vi "getPiezowaveformarray.vi"(7 "sawtooth or zigzag":bool, 8 "pixel.num":i32=10000, 9 "frames.per.z.cycle":dbl=15.0, 10 "total.z.distance":dbl=100.0, 11 "piezo scale factor":dbl=0.025) -> (3 "Array":dbl[](array[numeric]))   [LabVIEW 2017]
doc: "SciScan 1.2 160622"
uses:
  GFG/GFGnumericGet.vi
  GFG/GFG library.lvlib
panel:
  out "Waveform Graph":dbl[](graph)
  out "min value":dbl
  out "max value":dbl
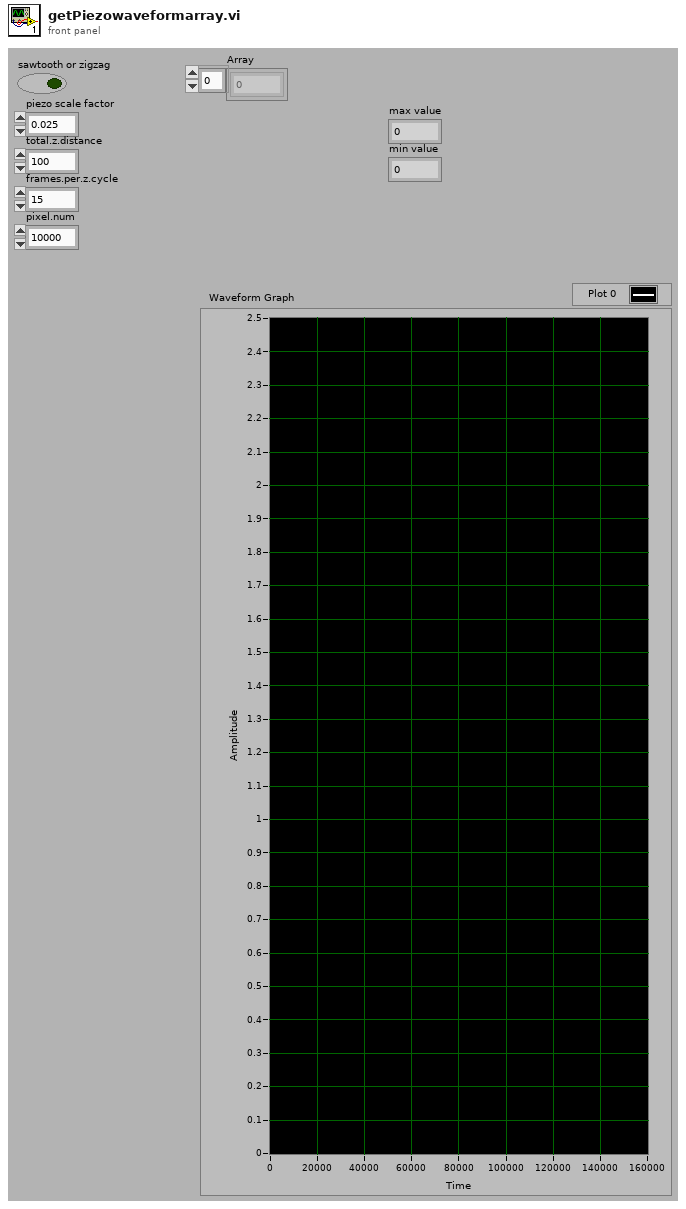
[diagram p1: front panel]
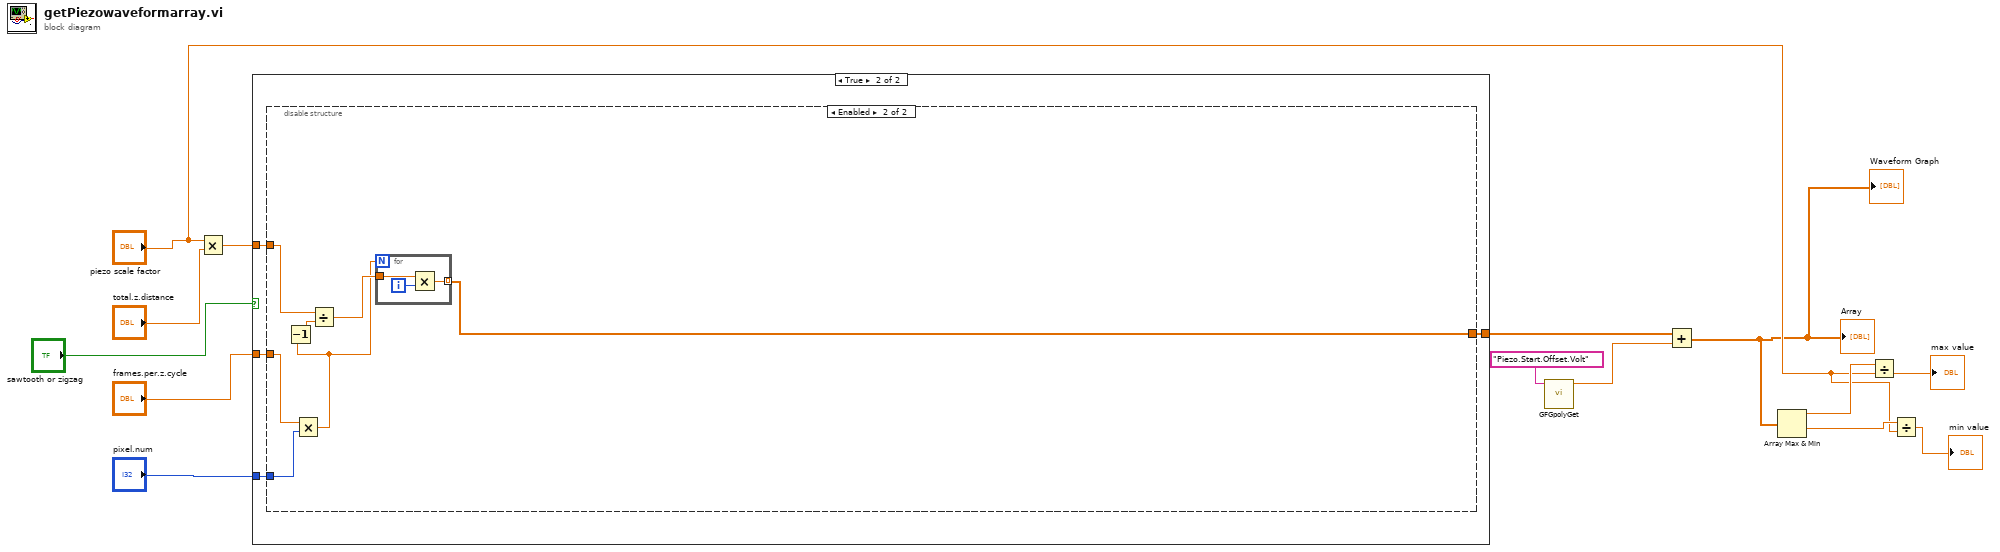
[diagram p0: block diagram]
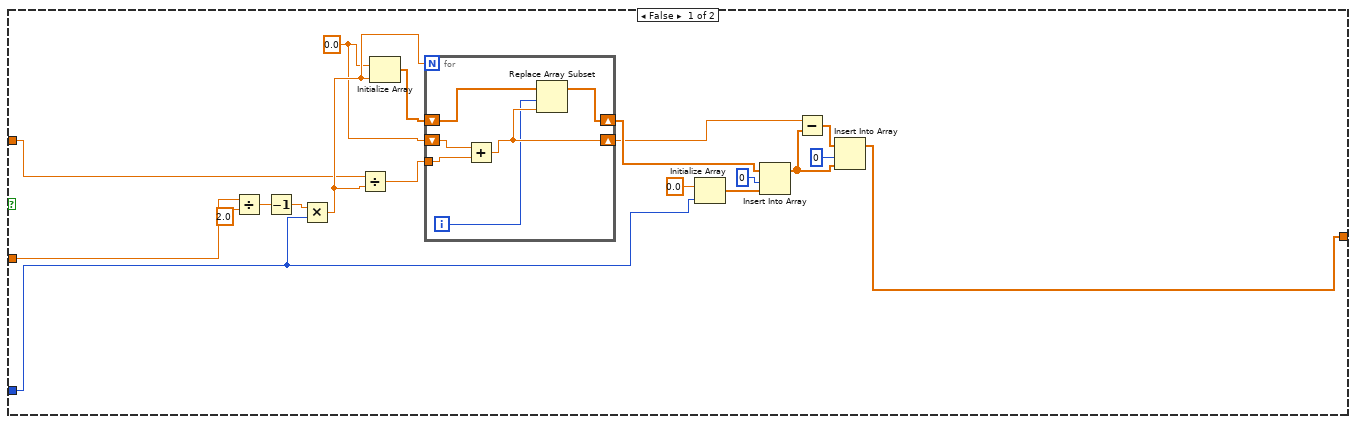
[diagram p2: hidden frame]
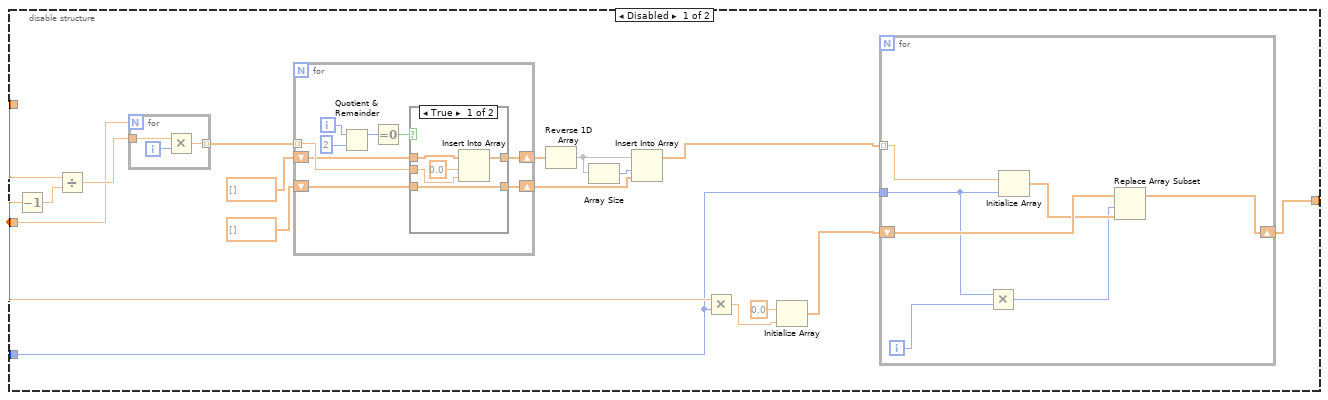
[diagram p3: hidden frame]
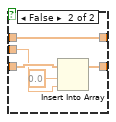
[diagram p4: hidden frame]
diagram:
  n1 = Multiply(x="piezo scale factor", y="total.z.distance") -> (x*y=w13:dbl)
  n2 = case shown="True" "sawtooth or zigzag" {
    tunnel: [w15 w43] -> w4
    tunnel: w13 -> [w18 w42]
    tunnel: "frames.per.z.cycle" -> [w17 w41]
    tunnel: "pixel.num" -> [w16 w40]
    frame False {
      w27 = 0.0 ("element")
      n3 = Divide(x=w17, y=2.0) -> (x/y=w32:dbl)
      n4 = Decrement(x=w32) -> (x-1=w31:dbl)
      n5 = Multiply(x=w31, y=w16) -> (x*y=w28:dbl)
      n6 = Divide(x=w18, y=w28) -> (x/y=w29:dbl)
      n7 = Initialize Array(w27, w28) -> (w30:dbl[])
      n8 = for {
        N: w28 -> [_]
        shift-right: [w36] -> w20
        shift-left: w30 -> [w37]
        tunnel: w29 -> [w38]
        shift-right: [w35] -> w19
        shift-left: w27 -> [w39]
        i -> [w34]
        n9 = Add(x=w39, y=w38) -> (x+y=w35:dbl)
        n10 = Replace Array Subset(array=w37, new element=w35, index=w34) -> (w36:dbl[])
      }
      n11 = Initialize Array(0.0 ("element"), w16) -> (w22:dbl[])
      n12 = Insert Into Array(array=w20, index=0, new element=w22) -> (w26:dbl[])
      n13 = Subtract(x=w19, y=w26) -> (x-y=w25:dbl[])
      n14 = Insert Into Array(array=w25, index=0, new element=w26) -> (w15:dbl[])
    }
    frame True {
      n15 = disable-structure shown="Enabled" {
        disable-tunnel: [w48 w90] -> w43
        disable-tunnel: w42 -> [w47 w95]
        disable-tunnel: w41 -> [w46 w94]
        disable-tunnel: w40 -> [w45 w93]
        frame Disabled {
          n16 = Decrement(x=w46) -> (x-1=w44:dbl)
          n17 = Divide(x=w47, y=w44) -> (x/y=w60:dbl)
          n18 = for {
            N: w46 -> [_]
            tunnel: w60 -> [w89]
            tunnel: [w87] -> w59 mode=indexing
            i -> [w88]
            n19 = Multiply(x=w89, y=w88) -> (x*y=w87:dbl)
          }
          n20 = for {
            shift-right: [w70] -> w55
            shift-left: dbl[] [] -> [w69]
            shift-right: [w71] -> w54
            shift-left: dbl[] [] -> [w72]
            tunnel: w59 -> [w74] mode=indexing
            i -> [w73]
            n21 = Quotient & Remainder(x=w73, y=2) -> (x-y*floor(x/y)=w68:i32)  [unwired: 1 out]
            n22 = Equal To 0?(x=w68) -> (x = 0?=w75:bool)
            n23 = case shown="True" w75 {
              tunnel: w74 -> [w77 w82]
              tunnel: w72 -> [w81 w83]
              tunnel: [w79 w83] -> w71
              tunnel: [w78 w84] -> w70
              tunnel: w69 -> [w78 w85]
              frame True {
                n24 = Insert Into Array(array=w81, index=0.0 ("new element/subarray"), new element=w77) -> (w79:dbl[])
              }
              frame False {
                n25 = Insert Into Array(array=w85, index=0.0 ("new element/subarray"), new element=w82) -> (w84:dbl[])
              }
            }
          }
          n26 = Reverse 1D Array(array=w54) -> (reversed array=w53:dbl[])
          n27 = Array Size(array=w53) -> (size(s)=w56:i32)
          n28 = Insert Into Array(array=w53, index=w56, new element=w55) -> (w52:dbl[])
          n29 = Multiply(x=w46, y=w45) -> (x*y=w49:dbl)
          n30 = Initialize Array(0.0 ("element"), w49) -> (w50:dbl[])
          n31 = for {
            tunnel: w52 -> [w67] mode=indexing
            shift-right: [w61] -> w48
            shift-left: w50 -> [w66]
            tunnel: w45 -> [w64]
            i -> [w63]
            n32 = Multiply(x=w64, y=w63) -> (x*y=w62:i32)
            n33 = Initialize Array(w67, w64) -> (w65:dbl[])
            n34 = Replace Array Subset(array=w66, new element=w65, index=w62) -> (w61:dbl[])
          }
        }
        frame Enabled {
          n35 = Multiply(x=w94, y=w93) -> (x*y=w91:dbl)
          n36 = Decrement(x=w91) -> (x-1=w92:dbl)
          n37 = Divide(x=w95, y=w92) -> (x/y=w96:dbl)
          n38 = for {
            N: w91 -> [_]
            tunnel: w96 -> [w99]
            tunnel: [w97] -> w90 mode=indexing
            i -> [w98]
            n39 = Multiply(x=w99, y=w98) -> (x*y=w97:dbl)
          }
        }
      }
    }
  }
  n40 = call-poly "GFGpolyGet.vi"("Variable Name in"="Piezo.Start.Offset.Volt") -> ("Numeric"=w1:dbl)  [unwired: 8 in, 2 out]
  n41 = Add(x=w4, y=w1) -> (x+y=w3:dbl[])
  "Array" <- w3
  "Waveform Graph" <- w3
  n42 = Array Max & Min(array=w3) -> (max value=w8:dbl, min value=w7:dbl)  [unwired: 2 out]
  n43 = Divide(x=w8, y="piezo scale factor") -> (x/y=→"max value":dbl)
  n44 = Divide(x=w7, y="piezo scale factor") -> (x/y=→"min value":dbl)
